vi "PluginsLoaderService_LoadPluginsForItem.vi"(8 "error in (no error)":errorcluster, 10 "ProjectItem":refnum<vi>, 11 "PluginsLoaderService in":refnum<class "PluginsLoaderService.lvclass">) -> (0 "error out":errorcluster, 3 "PluginsLoaderService out":refnum<class "PluginsLoaderService.lvclass">)   [LabVIEW 2014, in "PluginsThread.lvlib" / "PluginsLoaderService.lvclass"]
uses:
  PluginsLoaderService.lvclass
  _Plugins/GCMPlugin/GCMPlugin.lvclass
  PluginsLoaderService.lvclass/PluginsLoaderService.ctl
  _Plugins/_PluginLoader/_PluginLoader.lvclass
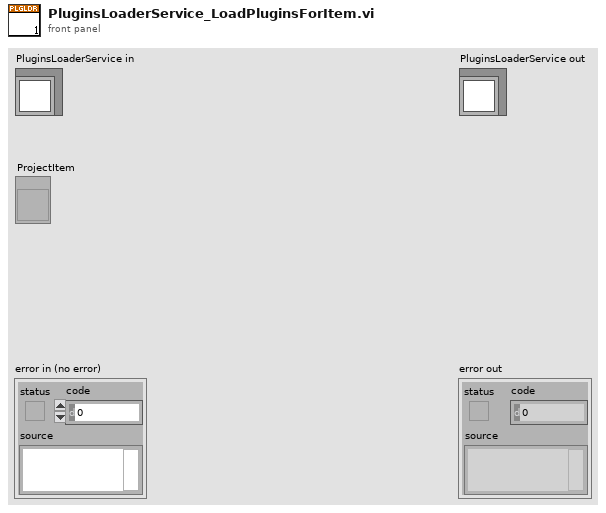
[diagram p1: front panel]
types:
  T1 = cluster{"CurrentItem":refnum<vi>, "AvailablePlugins":refnum<class "GCMPlugin.lvclass">[]}
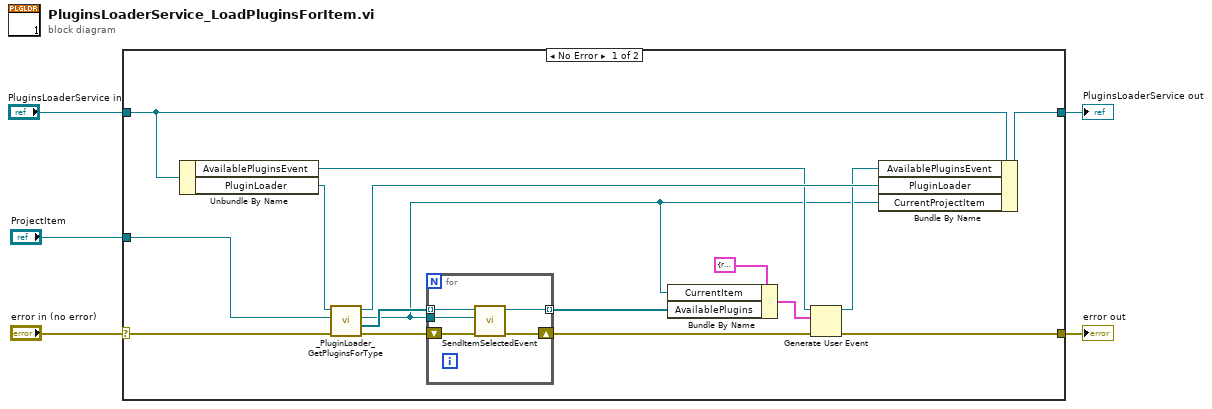
[diagram p0: block diagram]
diagram:
  n1 = case shown="No Error" "error in (no error)" {
    selector: "error in (no error)" -> [w20 w28]
    tunnel: [w19 w28] -> w4
    tunnel: [w16 w27] -> w2
    tunnel: "PluginsLoaderService in" -> [w18 w27]
    tunnel: "ProjectItem" -> [w21 _]
    frame No Error {
      n2 = Unbundle By Name(w18) -> ("AvailablePluginsEvent"=w14:refnum<user-event>, "PluginLoader"=w17:refnum<class "_PluginLoader.lvclass">)
      n3 = call "_PluginLoader_GetPluginsForType.vi"("error in (no error)"=w20, "ProjectItem"=w21, "_PluginLoader in"=w17) -> ("error out"=w9:errorcluster, "Plugins"=w10:refnum<class "GCMPlugin.lvclass">[], "ProjectItem out"=w6:refnum<vi>, "_PluginLoader out"=w15:refnum<class "_PluginLoader.lvclass">)  [unwired: 5 in]
      n4 = for {
        tunnel: w10 -> [w24] mode=indexing
        shift-right: [w22] -> w7
        shift-left: w9 -> [w26]
        tunnel: [w23] -> w8 mode=indexing
        tunnel: w6 -> [w25]
        n5 = call "SendItemSelectedEvent.vi"("error in (no error)"=w26, "ProjectItem"=w25, "_LVCMPlugin in"=w24) -> ("error out"=w22:errorcluster, "_LVCMPlugin out"=w23:refnum<class "GCMPlugin.lvclass">)  [unwired: 7 in]
      }
      n6 = Bundle By Name(cluster=T1 {"CurrentItem"=refnum, "AvailablePlugins"=[]} ("event data"), "CurrentItem"=w6, "AvailablePlugins"=w8) -> (w11:T1)
      n7 = Generate User Event(user event=w14, event data cluster=w11, error in=w7) -> (user event out=w13:refnum<user-event>, error out=w19:errorcluster)  [unwired: 1 in]
      n8 = Bundle By Name(cluster=w18, "AvailablePluginsEvent"=w13, "PluginLoader"=w15, "CurrentProjectItem"=w6) -> (w16:refnum<class "PluginsLoaderService.lvclass">)
    }
    frame Error {
    }
  }
  "error out" <- w4
  "PluginsLoaderService out" <- w2
